vi "GC ready status.vi"(0 "Serial Port":refnum<visa-resource-name>, 1 "switches":T3={"Oven"=TRUE, "Inj A heater"=TRUE, "Inj B heater"=TRUE, "Det A"=TRUE, "Det B"=FALSE, "Det A heater"=TRUE, "Det B heater"=FALSE}) -> (3 "oked":bool=TRUE, 4 "canceled":bool, 5 "Serial Port":refnum<visa-resource-name>, 6 "signals":enum16{"signal 1", "signals 1 and 2"}(ring)=enum."signals 1 and 2", 7 "Signal 1":T1, 8 "Det in use":string)   [LabVIEW 2012]
uses:
  signal.ctl
panel:
  out "Det B type":string
  out "Det A type":string
  out "?":T2={"Oven"=139.99, "Inj A"=200.0, "Inj B"=200.0, "Det A"=300.0, "Det B"=0.0} {"Inj B" scale=0.0..25.0 scale format="%.1f"; "Det B" scale=0.0..75.0 scale format="%.1f"; "Det A" scale=0.0..250.0 scale format="%.1f"; "Inj A" scale=0.0..250.0 scale format="%.1f"; "Oven" scale=0.0..100.0 scale format="%.1f"}
  out "Inj B set":sgl=200.0 format="%.1f"
  out "Det B set":sgl format="%.1f"
  out "Det A set":sgl=300.0 format="%.1f"
  out "Oven set":sgl=140.0 format="%.1f"
  out "Inj A set":sgl=200.0 format="%.1f"
  in  "cancel":bool
  in  "done":bool
  out "ramp":string=" "
  out "run status":T4(ring)
  out "Not Ready":T5
  # "Heater \non/off status"
  # "Detector status"
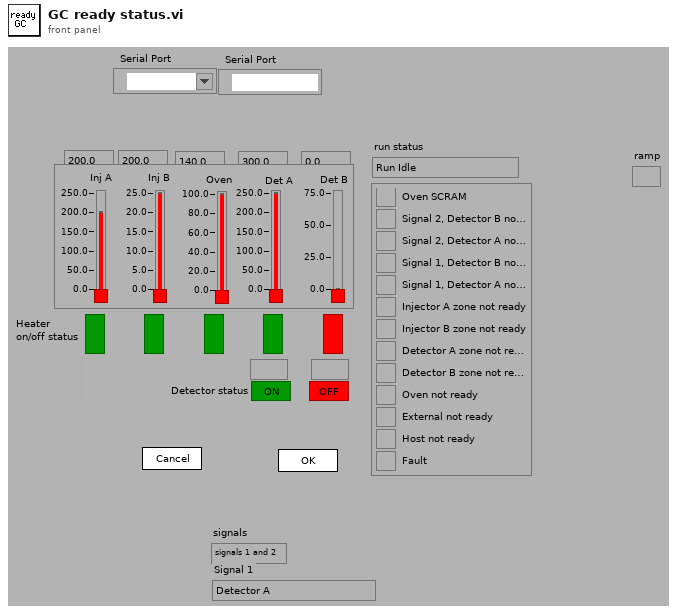
[diagram p1: front panel]
types:
  T1 = typedef "signal.ctl" = enum16{"Detector A", "Detector B", "Oven temperature", "Comp 1", "Comp 2", "Inlet A temperature", "Inlet B temperature", "Detector A temperature", "Detector B temperature", "Test Signal"}
  T2 = cluster{"Oven":dbl, "Inj A":dbl, "Inj B":dbl, "Det A":dbl, "Det B":dbl}
  T3 = cluster{"Oven":bool, "Inj A heater":bool, "Inj B heater":bool, "Det A":bool, "Det B":bool, "Det A heater":bool, "Det B heater":bool}
  T4 = enum16{"Run Idle", "Pre Run", "SCC Pre Run 1", "SCC Pre Run 2", "SCC Run", "Run Active", "Report 1", "Report 2", "Run Disabled (from outside GC)"}
  T5 = cluster{"Not used, always off":bool, "Not used, always off":bool, "Not used, always off":bool, "Oven SCRAM":bool, "Signal 2, Detector B not ON":bool, "Signal 2, Detector A not ON":bool, "Signal 1, Detector B not ON":bool, "Signal 1, Detector A not ON":bool, "Injector B zone not ready":bool, "Injector A zone not ready":bool, "Detector A zone not ready":bool, "Oven not ready":bool, "External not ready":bool, "Detector B zone not ready":bool, "Host not ready":bool, "Fault":bool}
  T6 = cluster{"Oven":bool, "Cryogenic":bool, "Inj. A Temp":bool, "Inj. B Temp":bool, "Det. A Temp":bool, "Det. B Temp":bool, "Signal 1 Zero":bool, "Signal 1 Attn.":bool, "Signal 2 Zero":bool, "Signal 2 Attn.":bool, "Det. A":bool, "Det. B":bool, "Purge A":bool, "Purge B":bool}
  T7 = cluster{"Version":sgl, "Initial Temp":sgl, "Oven On/Off":sgl, "Cryogenic  On/Off":sgl, "Oven Max":sgl, "Equib Time":sgl, "Initial Time":sgl, "Rate":dbl, "Final Temp":dbl, "Final Time":dbl, "Rate A":dbl, "Final Temp A":dbl, "Final Time A":dbl, "Rate B":dbl, "Final Temp B":dbl, "Final Time B":dbl, "Inj. A Temp":dbl, "Inj. A Temp On/Off":dbl, "Inj. B Temp":dbl, "Inj. B Temp On/Off":dbl, "Det. A Temp":dbl, "Det. A Temp On/Off":dbl, "Det. B Temp":dbl, "Det. B Temp On/Off":dbl, "Signal 1 Address":dbl, "Signal 1 Range":dbl, "Signal 1 Zero":dbl, "Signal 1 Zero On/Off":dbl, "Signal 1 Attn.":dbl, "Signal 1 Attn. On/Off":dbl, "Signal 2 Address":dbl, "Signal 2 Range":dbl, "Signal 2 Zero":dbl, "Signal 2 Zero On/Off":dbl, "Signal 2 Attn.":dbl, "Signal 2 Attn. On/Off":dbl, "Det. A On/Off":dbl, "Det. A Polarity":dbl, "Det. A Time":dbl, "Det. B On/Off":dbl, "Det. B Polarity":dbl, "Det. B Time":dbl, "Purge A On/Off":dbl, "Purge A On Time":dbl, "Purge A Off Time":dbl, "Purge B On/Off":dbl, "Purge B On Time":dbl, "Purge B Off Time":dbl}
  T8 = typedef "detector.ctl" = cluster{"Det A":string, "Det B":string}
  T9 = enum16{"Detector A", "Detector B", "Oven temperature", "Comp 1", "Comp 2", "Inlet A temperature", "Inlet B temperature", "Detector A temperature", "Detector B temperature", "Test Signal"}
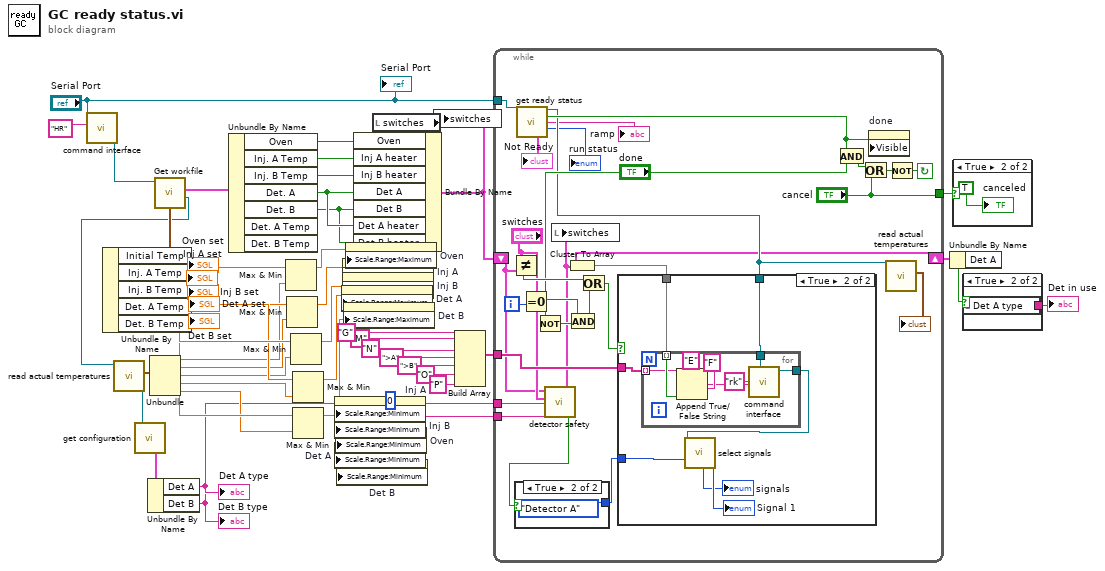
[diagram p0: block diagram]
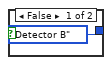
[diagram p2: hidden frame]
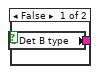
[diagram p4: hidden frame]
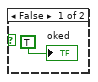
[diagram p5: hidden frame]
diagram:
  w35 = 0
  n1 = call "command interface.vi"("command"="HR", "Serial Port"="Serial Port") -> ("Serial Port"=w15:refnum<visa-resource-name>)  [unwired: 5 in, 3 out]
  n2 = call "Get workfile.vi"("Serial Port"=w15) -> ("Serial Port"=w14:refnum<visa-resource-name>, "On/Off status"=w46:T6, "Workfile"=w42:T7)  [unwired: 4 in]
  n3 = Unbundle By Name(w42) -> ("Initial Temp"=w30:sgl, "Inj. A Temp"=w29:dbl, "Inj. B Temp"=w34:dbl, "Det. A Temp"=w31:dbl, "Det. B Temp"=w32:dbl)
  "Inj A set" <- w29
  "Oven set" <- w30
  "Det A set" <- w31
  "Det B set" <- w32
  "Inj B set" <- w34
  n4 = call "read actual temperatures.vi"("Serial Port"=w14) -> (2:w33:T2, "Serial Port"=w9:refnum<visa-resource-name>)  [unwired: 4 in, 1 out]
  n5 = call "get configuration.vi"("Serial Port"=w9) -> ("Detectors"=w5:T8)  [unwired: 5 in, 2 out]
  n6 = Unbundle By Name(w5) -> ("Det A"=w4:string, "Det B"=w3:string)
  "Det A type" <- w4
  "Det B type" <- w3
  n7 = Unbundle(w33) -> ("Oven"=w28:dbl, "Inj A"=w27:dbl, "Inj B"=w26:dbl, "Det A"=w25:dbl, "Det B"=w23:dbl)
  n8 = Unbundle By Name(w46) -> ("Oven"=w39:bool, "Inj. A Temp"=w38:bool, "Inj. B Temp"=w37:bool, "Det. A"=w2:bool, "Det. B"=w1:bool)  [unwired: 2 out]
  n9 = Max & Min(x=w30, y=w28) -> (max(x,y)=w12:dbl)  [unwired: 1 out]
  n10 = Max & Min(x=w29, y=w27) -> (max(x,y)=w11:dbl)  [unwired: 1 out]
  n11 = Max & Min(x=w34, y=w26) -> (max(x,y)=w10:dbl)  [unwired: 1 out]
  n12 = Max & Min(x=w31, y=w25) -> (max(x,y)=w24:dbl)  [unwired: 1 out]
  n13 = Max & Min(x=w32, y=w23) -> (max(x,y)=w22:dbl)  [unwired: 1 out]
  n14 = property on="Inj A" class="Slide (strict)"("Scale.Range:Minimum"=w35) -> ()  [unwired: 2 in, 2 out]
  n15 = property on="Inj B" class="Slide (strict)"("Scale.Range:Minimum"=w35) -> ()  [unwired: 2 in, 2 out]
  n16 = property on="Det A" class="Slide (strict)"("Scale.Range:Minimum"=w35) -> ()  [unwired: 2 in, 2 out]
  n17 = property on="Oven" class="Slide (strict)"("Scale.Range:Minimum"=w35) -> ()  [unwired: 2 in, 2 out]
  n18 = property on="Det B" class="Slide (strict)"("Scale.Range:Minimum"=w35) -> ()  [unwired: 2 in, 2 out]
  n19 = property on="Det A" class="Slide (strict)"("Scale.Range:Maximum"=w24) -> ()  [unwired: 2 in, 2 out]
  n20 = property on="Inj A" class="Slide (strict)"("Scale.Range:Maximum"=w11) -> ()  [unwired: 2 in, 2 out]
  n21 = property on="Inj B" class="Slide (strict)"("Scale.Range:Maximum"=w10) -> ()  [unwired: 2 in, 2 out]
  n22 = property on="Det B" class="Slide (strict)"("Scale.Range:Maximum"=w22) -> ()  [unwired: 2 in, 2 out]
  n23 = property on="Oven" class="Slide (strict)"("Scale.Range:Maximum"=w12) -> ()  [unwired: 2 in, 2 out]
  n24 = local read "switches"() -> (w36:T3)
  n25 = Bundle By Name(cluster=w36, "Oven"=w39, "Inj A heater"=w38, "Inj B heater"=w37, "Det A"=w2, "Det B"=w1, "Det A heater"=w2, "Det B heater"=w1) -> (w40:T3)
  n26 = local write "switches"(w40) -> ()
  n27 = Build Array("G", "M", "N", ">A", ">B", "O", "P") -> (w43:string[])
  n28 = while {
    tunnel: w3 -> [w49]
    tunnel: w4 -> [w50]
    tunnel: ["cancel"] -> w41
    tunnel: w43 -> [w70]
    shift-left: w40 -> [w51]
    shift-right: [w47] -> w8
    tunnel: "Serial Port" -> [w60]
    i -> [w66]
    stop <- w71 continue-if-true
    n29 = Not Equal?(x="switches", y=w51) -> (x != y?=w68:bool)
    n30 = call "get ready status.vi"("Serial Port"=w60) -> ("Serial Port"=w59:refnum<visa-resource-name>, "ready"=w61:bool, "ramp"=→"ramp":string, "run status"=→"run status":T4, "Not Ready"=→"Not Ready":T5)  [unwired: 10 in]
    n31 = Equal To 0?(x=w66) -> (x = 0?=w63:bool)
    n32 = Not(x="done") -> (.not. x?=w64:bool)
    n33 = call "detector safety.vi"("Det B type"=w49, "Det A type"=w50, "switches in"="switches", "switches prev"=w51) -> ("Det A"=w48:bool, "switches out"=w47:T3)
    n34 = case shown="True" w48 {
      tunnel: [T9."Detector B" ("Signal 1") T9."Detector A" ("Signal 1")] -> w54
      frame False {
      }
      frame True {
      }
    }
    n35 = local write "switches"(w47) -> ()
    n36 = Cluster To Array(cluster=w47) -> (array=w53:bool[])
    n37 = And(x=w63, y=w64) -> (x .and. y?=w62:bool)
    n38 = Or(x=w68, y=w62) -> (x .or. y?=w67:bool)
    n39 = case shown="True" w67 {
      tunnel: w70 -> [_ w82]
      tunnel: w53 -> [_ w81]
      tunnel: w59 -> [_ w77]
      tunnel: w54 -> [_ w76]
      frame False {
      }
      frame True {
        n40 = for {
          tunnel: w82 -> [w86] mode=indexing
          tunnel: w81 -> [w88] mode=indexing
          tunnel: w77 -> [w84]
          tunnel: [w83] -> w78
          n41 = Append True/False String(1:w88, 2:"F", 3:"E", 4:w86) -> (0:w85:string)
          n42 = call "command interface.vi"("Parameter"=w85, "command"="rk", "Serial Port"=w84) -> ("Serial Port"=w83:refnum<visa-resource-name>)  [unwired: 4 in, 3 out]
        }
        n43 = call "select signals.vi"("Serial Port"=w78, "Signal 1"=w76) -> ("signals"=→"signals":enum16{"signal 1", "signals 1 and 2"}, "Signal 1"=→"Signal 1":T1)  [unwired: 10 in, 2 out]
      }
    }
    n44 = And(x=w61, y="done") -> (x .and. y?=w73:bool)
    n45 = Or(x=w73, y="cancel") -> (x .or. y?=w72:bool)
    n46 = property on="done" class="Bool"("Visible"=w61) -> ()  [unwired: 2 in, 2 out]
    n47 = call "read actual temperatures.vi"("Serial Port"=w59) -> (2:→"?":T2)  [unwired: 4 in, 2 out]
    n48 = Not(x=w72) -> (.not. x?=w71:bool)
  }
  n49 = Unbundle By Name(w8) -> ("Det A"=w7:bool)
  n50 = case shown="True" w41 {
    frame False {
      "oked" <- TRUE
    }
    frame True {
      "canceled" <- TRUE
    }
  }
  n51 = case shown="True" w7 {
    tunnel: [w93 w94] -> w6
    frame False {
      n52 = local read "Det B type"() -> (w93:string)
    }
    frame True {
      n53 = local read "Det A type"() -> (w94:string)
    }
  }
  "Det in use" <- w6
  "Serial Port" <- "Serial Port"
